vi "Read Authentication.vi"(8 "error in":errorcluster, 11 "DB-Engine in":refnum<class "DB-Interface.lvclass">) -> (0 "error out":errorcluster, 1 "Password":string, 2 "User":string, 3 "DB-Engine out":refnum<class "DB-Interface.lvclass">, 4 "Database":string)   [LabVIEW 2014, in "hse-db.lvlib" / "DB-Interface.lvclass"]
doc: "Returns the authentication data."
uses:
  DB-Interface.lvclass
  DB-Interface.lvclass/DB-Interface.ctl
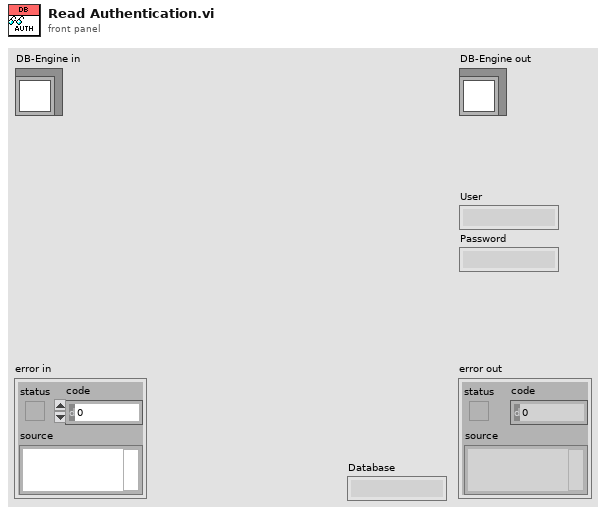
[diagram p1: front panel]
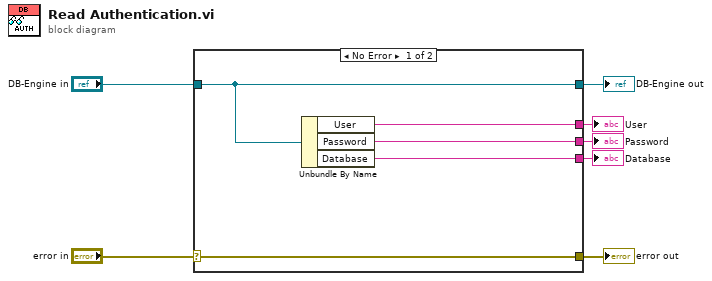
[diagram p0: block diagram]
diagram:
  n1 = case shown="No Error" "error in" {
    selector: "error in" -> [w12 w13]
    tunnel: [w12 w13] -> w6
    tunnel: [w11 w14] -> w4
    tunnel: "DB-Engine in" -> [w11 w14]
    tunnel: [w10 _] -> w3
    tunnel: [w9 _] -> w2
    tunnel: [w8 _] -> w1
    frame No Error {
      n2 = Unbundle By Name(w11) -> ("User"=w10:string, "Password"=w9:string, "Database"=w8:string)
    }
    frame Error {
    }
  }
  "error out" <- w6
  "DB-Engine out" <- w4
  "User" <- w3
  "Password" <- w2
  "Database" <- w1
